vi "GEOM_AddROIs.vi"(7 "Requested ROIs":T1, 9 "Corrrected ROIs":T1, 10 "amplifiers in":T3[](array[typedef]) {"fliped" items=["none", "horizontal", "vertical"]; "type" items=["LL", "LR", "UL", "UR"]}) -> (2 "amplifiers out":T3[](array[typedef]) {"fliped" items=["none", "horizontal", "vertical"]; "type" items=["LL", "LR", "UL", "UR"]})   [LabVIEW 2016]
uses:
  GEOM_Amplifier.ctl
  GEOM_AmpType.ctl
  GEOM_ROI.ctl
  GEOM_Coords.ctl
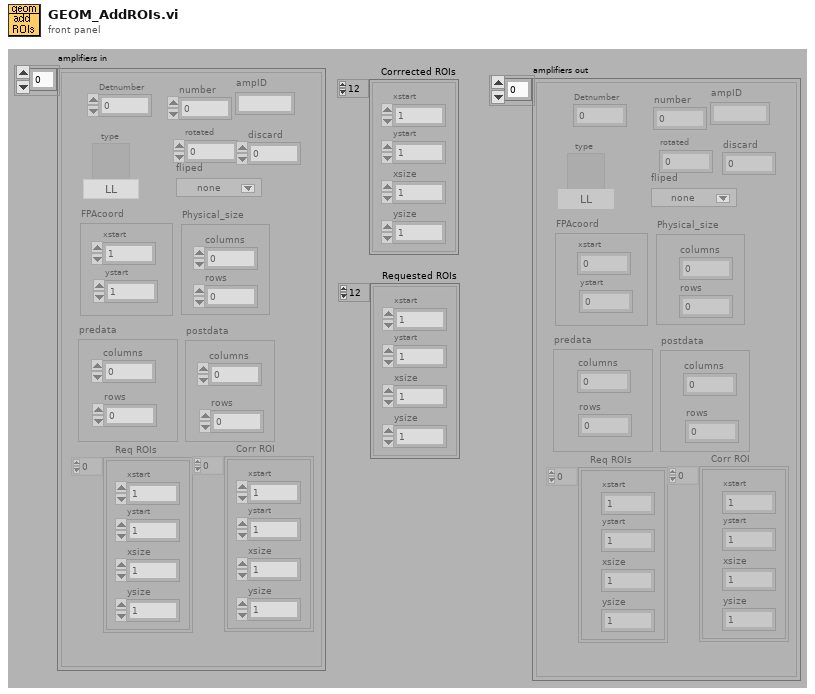
[diagram p1: front panel]
types:
  T1 = typedef "GEOM_ROI.ctl" = T2[]
  T2 = typedef "GEOM_Coords.ctl" = cluster{"xstart":u32, "ystart":u32, "xsize":u32, "ysize":u32}
  T3 = typedef "GEOM_Amplifier.ctl" = cluster{"number":i32, "type":T4, "rotated":i16, "fliped":u16, "FPAcoord":cluster{"xstart":i32, "ystart":i32}, "Physical_size":cluster{"columns":i32, "rows":i32}, "predata":cluster{"columns":i32, "rows":i32}, "postdata":cluster{"columns":i32, "rows":i32}, "Req ROIs":T1, "Corr ROI":T1, "Detnumber":i32, "ampID":string, "discard":i32}
  T4 = typedef "GEOM_AmpType.ctl" = u16
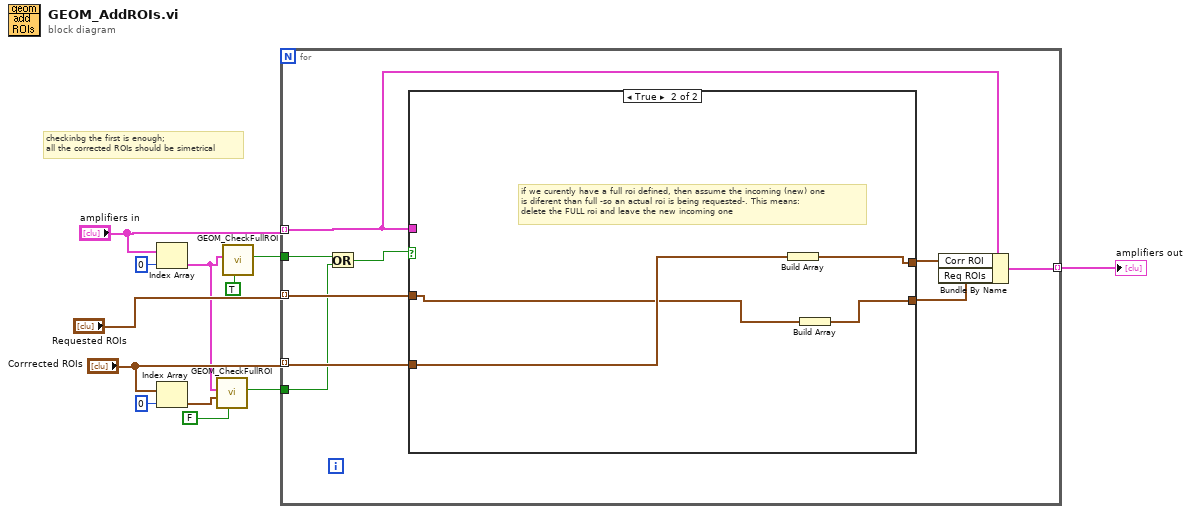
[diagram p0: block diagram]
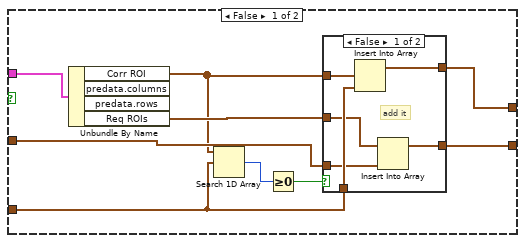
[diagram p2: hidden frame]
diagram:
  # "checkinbg the first is enough;\nall the corrected ROIs should be simetrical"
  n1 = Index Array(array="amplifiers in", index=0) -> (element=w5:T3)
  n2 = Index Array(array="Corrrected ROIs", index=0) -> (element=w4:T2)
  n3 = call "GEOM_CheckFullROI.vi"("self"=FALSE, "amproi"=w4, "Amplifier"=w5) -> ("full"=w2:bool)  [unwired: 8 out]
  n4 = call "GEOM_CheckFullROI.vi"("self"=TRUE, "Amplifier"=w5) -> ("full"=w1:bool)  [unwired: 1 in, 8 out]
  n5 = for {
    tunnel: "Corrrected ROIs" -> [w17] mode=indexing
    tunnel: "Requested ROIs" -> [w20] mode=indexing
    tunnel: "amplifiers in" -> [w16] mode=indexing
    tunnel: [w18] -> w11 mode=indexing
    tunnel: w2 -> [w13]
    tunnel: w1 -> [w15]
    n6 = Or(x=w15, y=w13) -> (x .or. y?=w14:bool)
    n7 = case shown="True" w14 {
      tunnel: [w30 w41] -> w21
      tunnel: w20 -> [w29 w39]
      tunnel: [w28 w42] -> w19
      tunnel: w17 -> [w23 w40]
      tunnel: w16 -> [w27 _]
      frame False {
        n8 = Unbundle By Name(w27) -> ("Corr ROI"=w22:T1, "Req ROIs"=w26:T1)  [unwired: 2 out]
        n9 = Search 1D Array(1D array=w22, element=w23) -> (index of element=w25:i32)  [unwired: 1 out]
        n10 = Greater Or Equal To 0?(x=w25) -> (x >= 0?=w24:bool)
        n11 = case shown="False" w24 {
          tunnel: w22 -> [w36 w38]
          tunnel: [w35 w38] -> w28
          tunnel: [w34 w37] -> w30
          tunnel: w23 -> [w33 _]
          tunnel: w26 -> [w32 w37]
          tunnel: w29 -> [w31 _]
          frame False {
            # "add it"
            n12 = Insert Into Array(array=w36, new element=w33) -> (w35:T1)  [unwired: 1 in]
            n13 = Insert Into Array(array=w32, new element=w31) -> (w34:T1)  [unwired: 1 in]
          }
          frame True {
            # "already there"
          }
        }
      }
      frame True {
        # "if we curently have a full roi defined, then assume the incoming (new) one\nis diferent than full -so an actual roi is being requested-. This means:\ndelete the FULL roi and leave the new incoming one"
        n14 = Build Array(w40) -> (w42:T2[])
        n15 = Build Array(w39) -> (w41:T2[])
      }
    }
    n16 = Bundle By Name(cluster=w16, "Corr ROI"=w19, "Req ROIs"=w21) -> (w18:T3)
  }
  "amplifiers out" <- w11
